vi "Flow Rate Value Unit to Register Data.vi"(0 "Flow Rate Value":dbl=100.0 caption="流量值", 3 "Flow Rate Unit":u16(ring)=2 caption="流量单位" items=["L/min", "mL/min", "uL/min", "nL/min"]) -> (7 "Valid Result":bool caption="有效结果？", 9 "Value Reg Data":dbl caption="值寄存器", 10 "Unit Reg Data":dbl caption="单位寄存器")   [LabVIEW 2023, in "Longer Pump dLSP501 Series.lvlib"]
uses:
  <instrlib>/Longer Pump dLSP501 Modbus RTU Series/Longer Pump dLSP501 Series.lvlib
panel:
  out "已强制转换(x)":dbl caption="强制转换结果"
  out "范围内？":bool caption="范围内 ?"
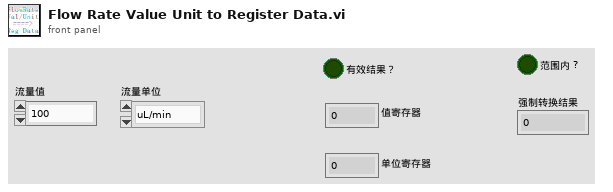
[diagram p1: front panel]
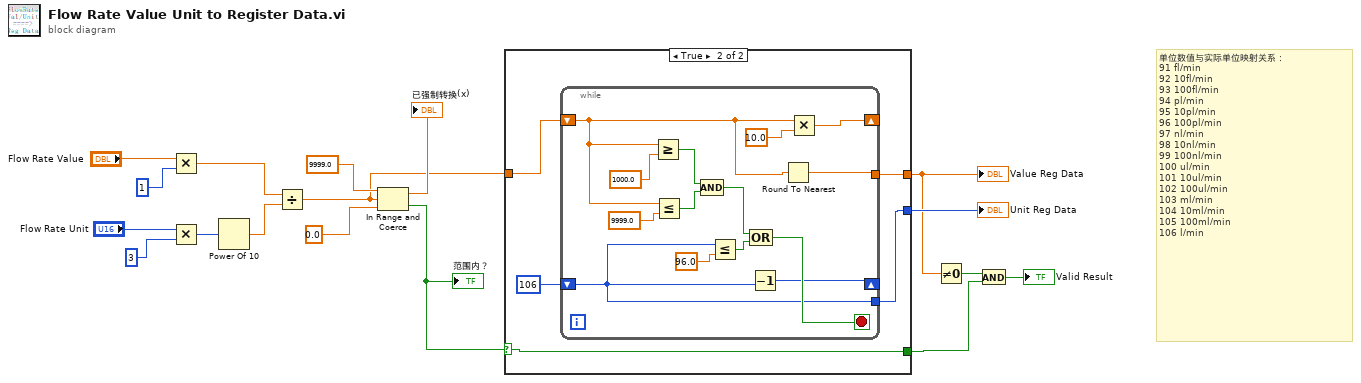
[diagram p0: block diagram]
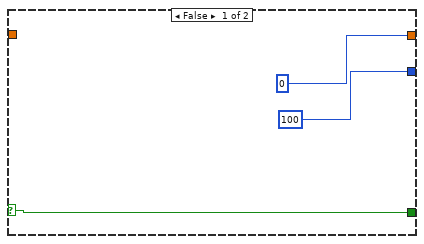
[diagram p2: hidden frame]
diagram:
  # "单位数值与实际单位映射关系：\n91\tfl/min\n92\t10fl/min\n93\t100fl/min\n94\tpl/min\n95\t10pl/min\n96\t100pl/min\n97\tnl/min\n98\t10nl/min\n99\t100nl/min\n100\tul/min\n101\t10ul/min\n102\t100ul/min\n103\tml/min\n104\t10ml/min\n105\t100ml/min\n106\tl/min"
  n1 = Multiply(x="Flow Rate Value", y=u16 1) -> (x*y=w12:dbl)
  n2 = Multiply(x="Flow Rate Unit", y=u16 3) -> (x*y=w15:u16)
  n3 = Power Of 10(x=w15) -> (10^x=w11:dbl)
  n4 = Divide(x=w12, y=w11) -> (x/y=w6:dbl)
  n5 = In Range and Coerce(upper limit=9999.0 ("x"), x=w6, lower limit=0.0 ("x")) -> (coerced(x)=→"已强制转换(x)":dbl, In Range?=w7:bool)
  "范围内？" <- w7
  n6 = case shown="True" w7 {
    selector: w7 -> [w20 w25]
    tunnel: w6 -> [_ w24]
    tunnel: [w20 w25] -> w3
    tunnel: [100 w21] -> w5
    tunnel: [0 w22] -> w2
    frame False {
    }
    frame True {
      n7 = while {
        shift-right: [w39] -> _
        shift-left: w24 -> [w27]
        shift-right: [w30] -> _
        shift-left: 106 -> [w28]
        tunnel: [w26] -> w22
        tunnel: [w28] -> w21
        stop <- w32 stop-if-true
        n8 = Greater Or Equal?(x=w27, y=1000.0 ("x")) -> (x >= y?=w35:bool)
        n9 = Less Or Equal?(x=w27, y=9999.0 ("x")) -> (x <= y?=w34:bool)
        n10 = Compound Arithmetic op=AND ("复合运算")(w35, w34) -> (w33:bool)
        n11 = Less Or Equal?(x=w28, y=96.0 ("x")) -> (x <= y?=w29:bool)
        n12 = Compound Arithmetic op=OR ("复合运算")(w33, w29) -> (w32:bool)
        n13 = Decrement(x=w28) -> (x-1=w30:i32)
        n14 = Round To Nearest(number=w27) -> (nearest integer value=w26:dbl)
        n15 = Multiply(x=w27, y=10.0) -> (x*y=w39:dbl)
      }
    }
  }
  "Value Reg Data" <- w2
  "Unit Reg Data" <- w5
  n16 = Not Equal To 0?(x=w2) -> (x != 0?=w4:bool)
  n17 = And(x=w4, y=w3) -> (x .and. y?=→"Valid Result":bool)
